vi "get_config_cluster.vi"(8 "error in (no error)":errorcluster, 11 "GenericPlugin in":refnum<class "StageMH110930Scientifica.lvclass">) -> (0 "error out":errorcluster, 2 "config cluster (variant)":variant, 3 "GenericPlugin out":refnum<class "StageMH110930Scientifica.lvclass">)   [LabVIEW 2010, in "StageMH110930Scientifica.lvclass"]
uses:
  StageMH110930Scientifica.lvclass
  StageMH110930Scientifica.lvclass/StageMH110930Scientifica.ctl
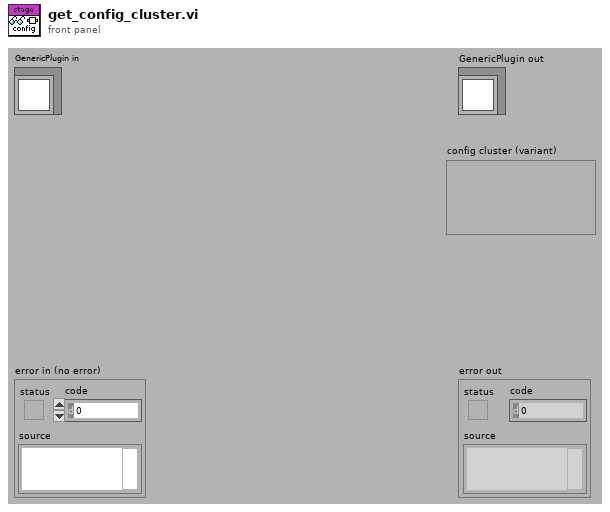
[diagram p1: front panel]
types:
  T1 = typedef "StageMH110930Scientifica.lvclass/config_data_cluster.ctl" = cluster{"serial port name":refnum<visa-resource-name>}
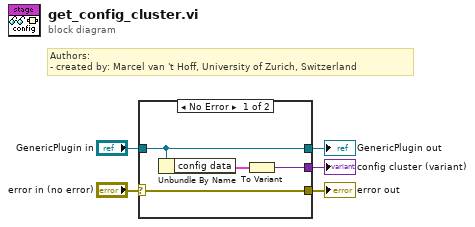
[diagram p0: block diagram]
diagram:
  # "Authors: \n- created by: Marcel van 't Hoff, University of Zurich, Switzerland"
  n1 = case shown="No Error" "error in (no error)" {
    selector: "error in (no error)" -> [w9 w10]
    tunnel: "GenericPlugin in" -> [w8 w11]
    tunnel: [w9 w10] -> w3
    tunnel: [w8 w11] -> w2
    tunnel: [w6 _] -> w1
    frame No Error {
      n2 = Unbundle By Name(w8) -> ("config data"=w7:T1)
      n3 = To Variant(anything=w7) -> (Variant=w6:variant)
    }
    frame Error {
    }
  }
  "error out" <- w3
  "GenericPlugin out" <- w2
  "config cluster (variant)" <- w1
